vi "Read Spec Page Path.vi"(8 "error in (no error)":errorcluster, 11 "MLUG in":refnum<class "MLUG.lvclass">) -> (0 "error out":errorcluster, 2 "Path to Spec Page VI":path, 3 "MLUG out":refnum<class "MLUG.lvclass">)   [LabVIEW 2020, in "MLUG.lvclass"]
uses:
  MLUG.lvclass
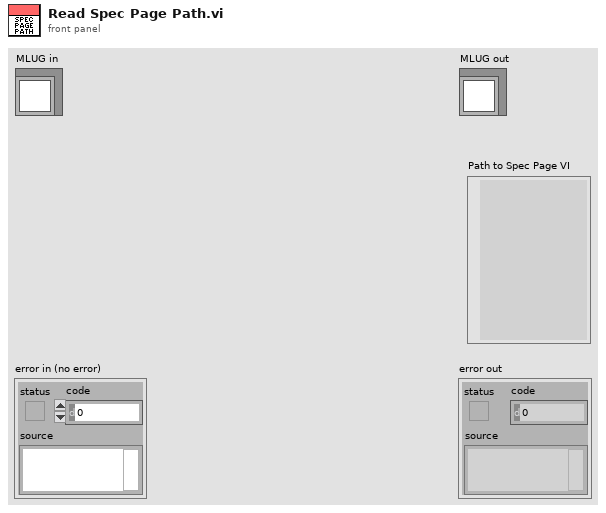
[diagram p1: front panel]
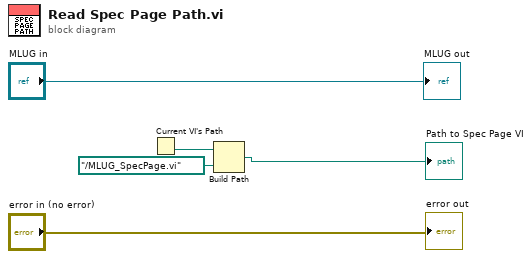
[diagram p0: block diagram]
diagram:
  n1 = Current VI's Path() -> (path=w4:path)
  n2 = Build Path(base path=w4, name or relative path=path "../MLUG_SpecPage.vi") -> (appended path=→"Path to Spec Page VI":path)
  "error out" <- "error in (no error)"
  "MLUG out" <- "MLUG in"
